vi "Write Case-Controller Msg.vi"(10 "UserConsole.lvlib:Case-Controller Msg.lvclass":refnum<class "Case-Controller Msg.lvclass">, 11 "UserConsole in":refnum<class "UserConsole.lvclass">) -> (3 "UserConsole out":refnum<class "UserConsole.lvclass">)   [LabVIEW 2025, in "UserConsole.lvlib" / "UserConsole.lvclass"]
uses:
  UserConsole.lvclass
  UserConsole Messages/Case-Controller Msg/Case-Controller Msg.lvclass
  UserConsole.lvclass/UserConsole.ctl
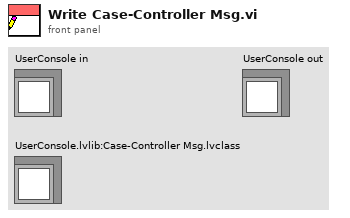
[diagram p1: front panel]
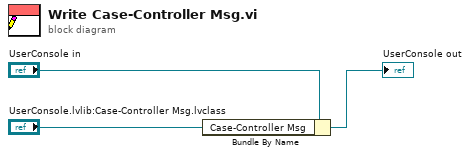
[diagram p0: block diagram]
diagram:
  n1 = Bundle By Name(cluster="UserConsole in", "Case-Controller Msg"="UserConsole.lvlib:Case-Controller Msg.lvclass") -> (→"UserConsole out":refnum<class "UserConsole.lvclass">)
